vi "Node - Update Reader Ch Values.vi"(8 "error in (no error)":errorcluster, 11 "Node Data In":T1) -> (0 "error out":errorcluster, 2 "Reader Ch Out":dbl[](array[numeric]), 3 "Node Data Out":T1)   [LabVIEW 2016, in "PXImc Router.lvlib"]
uses:
  PXImc Router.lvlib
  Controls/Node Data.ctl
  <vilib>/NI Veristand/VeriStand Data/Byte Buffer/Byte Buffer.lvclass
  Controls/Node/Node - PXImc Parameters.ctl
  Controls/Node/Transfer Data.ctl
  Controls/Node/Node Ch Properties.ctl
  Controls/Data Type.ctl
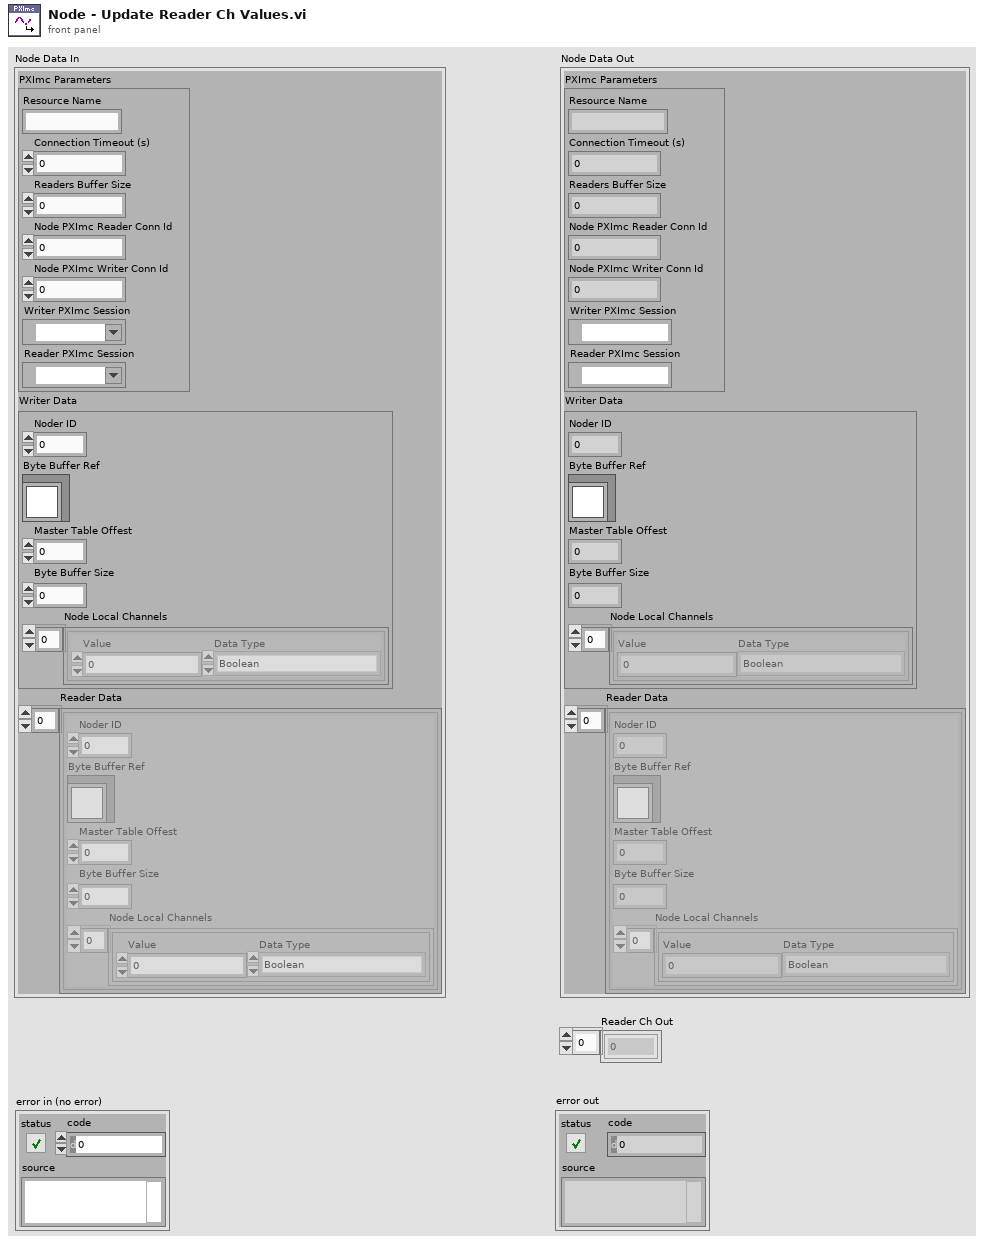
[diagram p1: front panel]
types:
  T1 = typedef "PXImc Router.lvlib/Node Data.ctl" = cluster{"PXImc Parameters":T2, "Writer Data":T3, "Reader Data":T3[]}
  T2 = typedef "PXImc Router.lvlib/Node - PXImc Parameters.ctl" = cluster{"Resource Name":string, "Connection Timeout (s)":dbl, "Readers Buffer Size":u64, "Node PXImc Reader Conn Id":u16, "Node PXImc Writer Conn Id":u16, "Writer PXImc Session":refnum<k21>, "Reader PXImc Session":refnum<k21>}
  T3 = typedef "PXImc Router.lvlib/Transfer Data.ctl" = cluster{"Noder ID":u32, "Byte Buffer Ref":refnum<class "Byte Buffer.lvclass">, "Master Table Offest":u32, "Byte Buffer Size":u32, "Node Local Channels":T4[]}
  T4 = typedef "PXImc Router.lvlib/Node Ch Properties.ctl" = cluster{"Value":dbl, "Data Type":T5}
  T5 = typedef "PXImc Router.lvlib/Data Type.ctl" = enum16{"Boolean", "SGL", "DBL", "I8", "I16", "I32", "I64", "U8", "U16", "U32", "U64"}
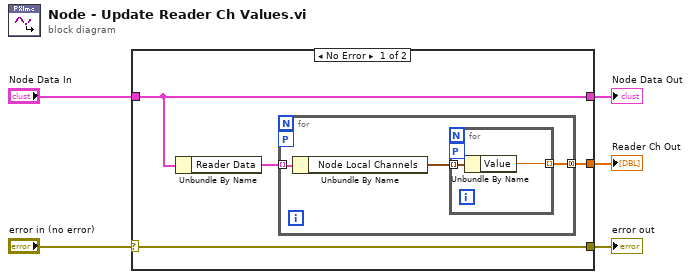
[diagram p0: block diagram]
diagram:
  n1 = case shown="No Error" "error in (no error)" {
    selector: "error in (no error)" -> [w8 w15]
    tunnel: "Node Data In" -> [w7 w16]
    tunnel: [w7 w16] -> w3
    tunnel: [w8 w15] -> w2
    tunnel: [w6 _] -> w1
    frame No Error {
      n2 = Unbundle By Name(w7) -> ("Reader Data"=w9:T3[])
      n3 = for {
        tunnel: w9 -> [w12] mode=indexing
        workers-P: _ -> [_]
        tunnel: [w10] -> w6 mode=concatenating
        n4 = Unbundle By Name(w12) -> ("Node Local Channels"=w11:T4[])
        n5 = for {
          tunnel: w11 -> [w14] mode=indexing
          tunnel: [w13] -> w10 mode=indexing
          workers-P: _ -> [_]
          n6 = Unbundle By Name(w14) -> ("Value"=w13:dbl)
        }
      }
    }
    frame Error {
    }
  }
  "Node Data Out" <- w3
  "error out" <- w2
  "Reader Ch Out" <- w1
